vi "csm_lumikki_instron_moveToSetpoint_2.vi"(7 "channelInt":i32=1, 8 "rampRate":dbl=1.0, 9 "rampAmplitude":dbl=1.0, 10 "setPointTime":dbl=1.0, 11 "setPoint":dbl=1.0) -> (3 "setPointOut":dbl=1.0)   [LabVIEW 2009]
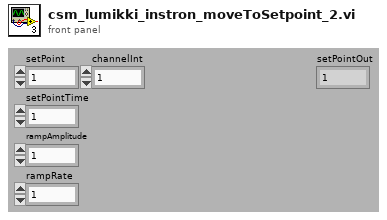
[diagram p1: front panel]
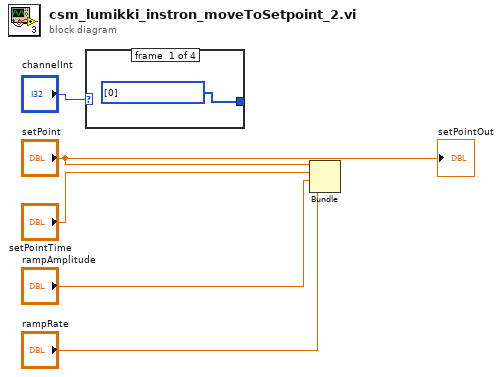
[diagram p0: block diagram]
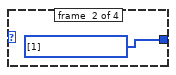
[diagram p2: hidden frame]
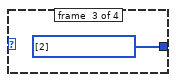
[diagram p3: hidden frame]
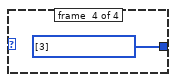
[diagram p4: hidden frame]
diagram:
  n1 = case shown="4" "channelInt" {
    tunnel: [w6 w7 w8 w9] -> _
    frame #0 {
      w6 = u16[] [0] items=["Channel 1", "Channel 2", "Channel 3", "Channel 4"] ("Choose channel to apply\nthe setpoint")
    }
    frame #1 {
      w7 = u16[] [1] items=["Channel 1", "Channel 2", "Channel 3", "Channel 4"] ("Choose channel to apply\nthe setpoint")
    }
    frame #2 {
      w8 = u16[] [2] items=["Channel 1", "Channel 2", "Channel 3", "Channel 4"] ("Choose channel to apply\nthe setpoint")
    }
    frame #3 {
      w9 = u16[] [3] items=["Channel 1", "Channel 2", "Channel 3", "Channel 4"] ("Choose channel to apply\nthe setpoint")
    }
  }
  n2 = Bundle("setPoint"="setPoint", "setPointTime"="setPointTime", "rampAmplitude"="rampAmplitude", "rampRate"="rampRate") -> ()  [unwired: 1 in, 1 out]
  "setPointOut" <- "setPoint"
